vi "Write writeRDs.vi"(8 "error in":errorcluster, 10 "Write?":bool, 11 "CRDS in":refnum<class "CRDS.lvclass">=refnum) -> (0 "error out":errorcluster, 3 "CRDS out":refnum<class "CRDS.lvclass">)   [LabVIEW 2014, in "CRDS.lvclass"]
uses:
  CRDS.lvclass
  Session APIs/Session Log/System Log.lvclass
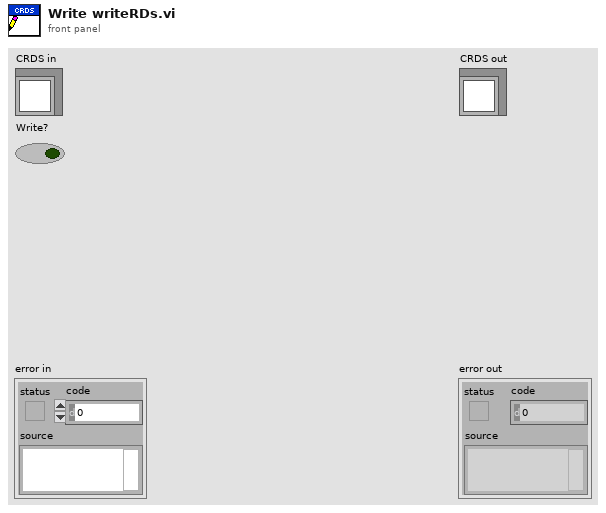
[diagram p1: front panel]
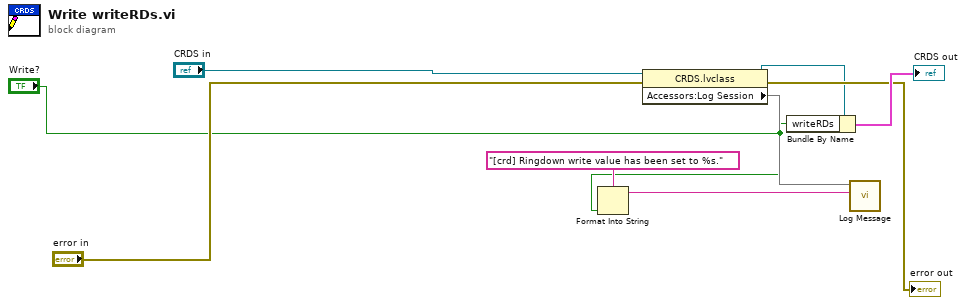
[diagram p0: block diagram]
diagram:
  n1 = Format Into String(format string="[crd] Ringdown write value has been set to %s.", "Write?") -> (resulting string=w3:string)  [unwired: 2 in, 1 out]
  n2 = property class="CRDS.lvclass"(reference="CRDS in", error in="error in") -> (reference out=w5:refnum<class "CRDS.lvclass">, error out=→"error out":errorcluster, "Accessors:Log Session"=w2)
  n3 = Bundle By Name(cluster=w5, "writeRDs"="Write?") -> (→"CRDS out":cluster{})
  n4 = call "Log Message.vi"("MSG In"=w3, "session in"=w2) -> ()  [unwired: 8 in, 2 out]
